vi "MICS_Channel Global.vi"() -> ()   [LabVIEW 2020]
panel:
  in  "MICS Channel":u16
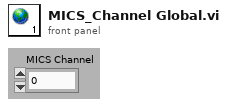
[diagram p1: front panel]
diagram:
